vi "MC Status.vi"() -> (2 "Subsystem Status":T1)   [LabVIEW 2015]
uses:
  Subsystem Status.ctl
  Subsystem Status Severity.ctl
  Subsystem Status Message.ctl
  Global Data.vi
panel:
  in  "Warm Motor Threshold":dbl=90.0
  in  "Warm MC Threshold":dbl=90.0
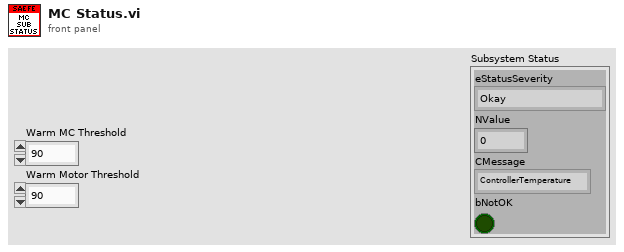
[diagram p1: front panel]
types:
  T1 = typedef "Subsystem Status.ctl" = cluster{"eStatusSeverity":T2, "NValue":sgl, "CMessage":T3, "bNotOK":bool}
  T2 = typedef "Subsystem Status Severity.ctl" = enum16{"Okay", "Short Warning", "Long Warning", "Return to Pits", "Error", "Danger"}
  T3 = typedef "Subsystem Status Message.ctl" = enum16{"ControllerTemperature", "MotorTemperature", "BatteryTemperature", "BatteryLowVoltage", "LVBattery", "sbRIOTemperature", "Precharge", "BSPD", "IMD", "RemoteReturnToPits", "EStopInterrupted", "NoCellComms", "MCOverSpeed", "MCOverCurrent", "MCOverVoltage", "MCInverterOverTemp", "MCDirectionCommand", "MCInverterTimeout", "MCDesatFault", "MCHWOverCurrent", "MCUnderVoltage", "MCCommandMessageLost", "MotorOverTemp", "MCModAOverTemp", "MCModBOverTemp", "MCModCOverTemp", "MCPCBOverTemp", "MCGateDrv1OverTemp", "MCDateDrv2OverTemp", "MCCurrentSensorFault", "MCResolverNotConnected", "ShutdownLatchTripped", "UnknownBMS", "RemoteEmergency"}
  T4 = typedef "MC Temp 1.ctl" = cluster{"TMCModuleA":dbl, "TMCModuleB":dbl, "TMCModuleC":dbl, "TMCGateDriver":dbl}
  T5 = typedef "MC Temp 2.ctl" = cluster{"TMCControlBoard":dbl, "TMCRTD1":dbl, "TMCRTD2":dbl, "TMCRTD3":dbl}
  T6 = typedef "MC Faults.ctl" = cluster{"MC Fault":cluster{"Over-Speed":bool, "Over-Current":bool, "Over-Voltage":bool, "Inverter Over-Temp":bool, "Direction Command":bool, "Inverter Response Time-Out":bool, "Desat Fault":bool, "Hardware Over-Current":bool, "Under-Voltage":bool, "CAN Command Message Lost":bool, "Motor Over-Temp":bool, "Module A Over-Temp":bool, "Module B Over-Temp":bool, "Module C Over-Temp":bool, "PCB Over-Temp":bool, "Gate Driver 1 Over-Temp":bool, "Gate Driver 2 Over-Temp":bool, "Gate Drive 3 Over-Temp":bool, "Current Sensor Fault":bool, "Resolver Not Connected":bool}, "MC Post":u32, "MC RUN":u32}
  T7 = cluster{"Over-Speed":bool, "Over-Current":bool, "Over-Voltage":bool, "Inverter Over-Temp":bool, "Direction Command":bool, "Inverter Response Time-Out":bool, "Desat Fault":bool, "Hardware Over-Current":bool, "Under-Voltage":bool, "CAN Command Message Lost":bool, "Motor Over-Temp":bool, "Module A Over-Temp":bool, "Module B Over-Temp":bool, "Module C Over-Temp":bool, "PCB Over-Temp":bool, "Gate Driver 1 Over-Temp":bool, "Gate Driver 2 Over-Temp":bool, "Gate Drive 3 Over-Temp":bool, "Current Sensor Fault":bool, "Resolver Not Connected":bool}
  T8 = typedef "MC Temp 3.ctl" = cluster{"TMCRTD4":dbl, "TMCRTD5":dbl, "TMotor":dbl, "MTorqueShudder":dbl}
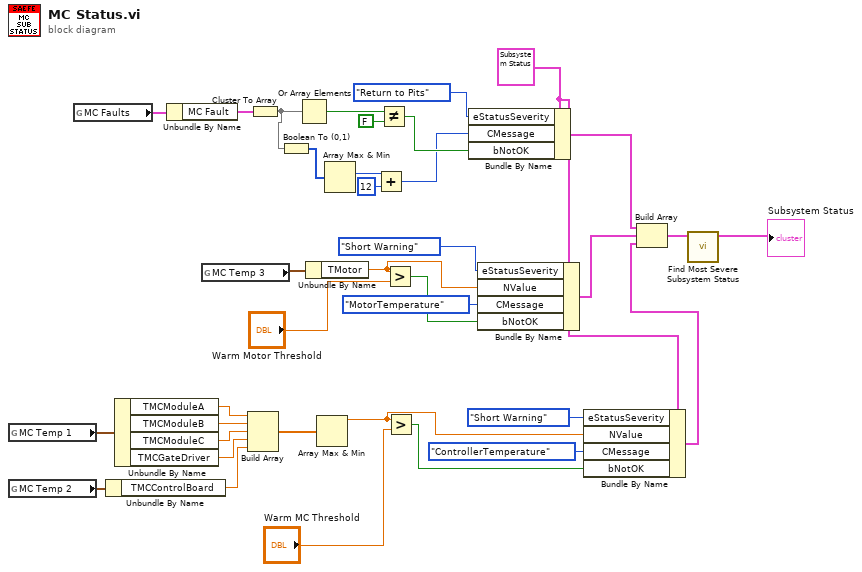
[diagram p0: block diagram]
diagram:
  w6 = T1 {"eStatusSeverity"=enum."Okay", "NValue"=0.0, "CMessage"=enum."ControllerTemperature", "bNotOK"=FALSE} ("Subystem Status")
  n1 = global read "Global Data.vi" "MC Temp 1"() -> (w33:T4)
  n2 = global read "Global Data.vi" "MC Temp 2"() -> (w32:T5)
  n3 = global read "Global Data.vi" "MC Faults"() -> (w31:T6)
  n4 = Unbundle By Name(w32) -> ("TMCControlBoard"=w22:dbl)
  n5 = Unbundle By Name(w33) -> ("TMCModuleA"=w27:dbl, "TMCModuleB"=w26:dbl, "TMCModuleC"=w25:dbl, "TMCGateDriver"=w24:dbl)
  n6 = Unbundle By Name(w31) -> ("MC Fault"=w30:T7)
  n7 = global read "Global Data.vi" "MC Temp 3"() -> (w34:T8)
  n8 = Build Array(w27, w26, w25, w24, w22) -> (w23:dbl[])
  n9 = Cluster To Array(cluster=w30) -> (array=w20:bool[])
  n10 = Boolean To (0,1)(Boolean=w20) -> (0, 1=w19:i16[])
  n11 = Or Array Elements(Boolean array=w20) -> (logical OR=w29:bool)
  n12 = Unbundle By Name(w34) -> ("TMotor"=w9:dbl)
  n13 = Array Max & Min(array=w23) -> (max value=w3:dbl)  [unwired: 3 out]
  n14 = Array Max & Min(array=w19) -> (max index (indices)=w18:i32)  [unwired: 3 out]
  n15 = Add(x=w18, y=12) -> (x+y=w16:i32)
  n16 = Not Equal?(x=w29, y=FALSE) -> (x != y?=w21:bool)
  n17 = Greater?(x=w9, y="Warm Motor Threshold") -> (0:w10:bool)
  n18 = Greater?(x=w3, y="Warm MC Threshold") -> (0:w5:bool)
  n19 = Bundle By Name(cluster=w6, "eStatusSeverity"=Subsystem_Status_Severity."Return to Pits" ("Status Severity"), "CMessage"=w16, "bNotOK"=w21) -> (w12:T1)
  n20 = Bundle By Name(cluster=w6, "eStatusSeverity"=Subsystem_Status_Severity."Short Warning" ("Status Severity"), "NValue"=w9, "CMessage"=Subsystem_Status_Message."MotorTemperature" ("Message"), "bNotOK"=w10) -> (w7:T1)
  n21 = Bundle By Name(cluster=w6, "eStatusSeverity"=Subsystem_Status_Severity."Short Warning" ("Status Severity"), "NValue"=w3, "CMessage"=Subsystem_Status_Message."ControllerTemperature" ("Message"), "bNotOK"=w5) -> (w1:T1)
  n22 = Build Array(w12, w7, w1) -> (w13:T1[])
  n23 = call "Find Most Severe Subsystem Status.vi"("Array"=w13) -> ("Subystem Status"=→"Subsystem Status":T1)  [unwired: 10 in]
